vi "log analysis_gps.vi"() -> ()   [LabVIEW 2019] (continued)
,0*ce1f2ed1\n\t", "DUALANTENNAHEADINGA,USB3,0,53.0,FINESTEERING,2107,282441.200,02000000,d426,15824;SOL_COMPUTED,L1_FLOAT,-1.000000000,98.119506836,-70.068420410,0.0,360.000000000,180.000000000,\"631T\",15,6,6,6,04,00,20,02*34737370\n\t", "INSPVAXA,USB3,0,53.0,FINESTEERING,2107,282441.700,02000000,471d,15824;INS_ALIGNMENT_COMPLETE,INS_RTKFIXED,37.37044907161,126.72457798223,11.5726,22.3000,-0.1948,0.2179,0.0112,0.019648441,1.409240811,126.353403085,0.4397,0.2935,0.5431,0.1139,0.0925,0.0768,0.1391,0.1441,5.0591,0f000001,0*4c7348f3\n\t", "DUALANTENNAHEADINGA,USB3,0,53.0,FINESTEERING,2107,282442.200,02000000,d426,15824;SOL_COMPUTED,L1_FLOAT,-1.000000000,135.735549927,-62.905853271,0.0,360.000000000,180.000000000,\"631T\",15,6,6,6,04,00,20,02*7d1a323e\n\t", "DUALANTENNAHEADINGA,USB3,0,53.0,FINESTEERING,2107,282442.700,02000000,d426,15824;SOL_COMPUTED,L1_FLOAT,-1.000000000,139.850036621,-63.364013672,0.0,360.000000000,180.000000000,\"631T\",16,6,6,6,04,00,20,02*201824d6\n\t", "INSPVAXA,USB3,0,51.0,FINESTEERING,2107,282443.200,02000000,471d,15824;INS_ALIGNMENT_COMPLETE,INS_RTKFIXED,37.37044646413,126.72458151712,11.5864,22.3000,-0.1973,0.2015,0.0164,-0.221608077,1.394071169,127.627895652,0.4382,0.2942,0.5425,0.1139,0.0929,0.0768,0.1390,0.1440,5.0619,0f000001,0*d0821dfc\n\t", "DUALANTENNAHEADINGA,USB3,0,51.0,FINESTEERING,2107,282443.700,02000000,d426,15824;SOL_COMPUTED,NARROW_FLOAT,-1.000000000,112.599952698,-57.933044434,0.0,360.000000000,180.000000000,\"631T\",15,6,6,6,04,00,20,03*0a41350b\n\t", "DUALANTENNAHEADINGA,USB3,0,52.5,FINESTEERING,2107,282444.200,02000000,d426,15824;SOL_COMPUTED,L1_FLOAT,-1.000000000,94.401931763,-65.202850342,0.0,360.000000000,180.000000000,\"631T\",17,6,6,6,04,00,20,03*e210f1e8\n\t", "INSPVAXA,USB3,0,52.5,FINESTEERING,2107,282444.700,02000000,471d,15824;INS_ALIGNMENT_COMPLETE,INS_RTKFIXED,37.37044378367,126.72458489519,11.6040,22.3000,-0.1971,0.2104,0.0118,-0.197880099,2.000562987,128.752453378,0.4375,0.2942,0.5421,0.1140,0.0930,0.0767,0.1389,0.1439,5.0634,0f000001,0*c33b9934\n\t", "INSPVAXA,USB3,0,52.0,FINESTEERING,2107,282445.200,02000000,471d,15824;INS_ALIGNMENT_COMPLETE,INS_RTKFIXED,37.37044286692,126.72458603367,11.6088,22.3000,-0.1958,0.2105,0.0125,-0.182257004,1.882197193,129.119511082,0.4372,0.2942,0.5419,0.1140,0.0930,0.0767,0.1387,0.1438,5.0651,0f000001,0*e6286548\n\t", "INSPVAXA,USB3,0,52.0,FINESTEERING,2107,282445.700,02000000,471d,15824;INS_ALIGNMENT_COMPLETE,INS_RTKFIXED,37.37044196596,126.72458716165,11.6139,22.3000,-0.1860,0.1986,0.0135,-0.288793449,1.691261499,129.571848658,0.4372,0.2942,0.5419,0.1140,0.0930,0.0767,0.1387,0.1438,5.0651,0f000001,0*93ea3f3c\n\t", "INSPVAXA,USB3,0,49.5,FINESTEERING,2107,282446.200,02000000,471d,15824;INS_ALIGNMENT_COMPLETE,INS_RTKFIXED,37.37044104802,126.72458827290,11.6191,22.3000,-0.2036,0.2086,0.0326,-0.314944845,1.597002545,130.029060418,0.4370,0.2950,0.5417,0.1141,0.0931,0.0767,0.1386,0.1437,5.0666,0f000001,0*166a3618\n\t", "DUALANTENNAHEADINGA,USB3,0,49.5,FINESTEERING,2107,282446.700,02000000,d426,15824;SOL_COMPUTED,L1_FLOAT,-1.000000000,72.571334839,-68.740661621,0.0,360.000000000,180.000000000,\"631T\",16,6,6,6,04,00,20,02*f8abca53\n\t", "DUALANTENNAHEADINGA,USB3,0,51.0,FINESTEERING,2107,282447.200,02000000,d426,15824;SOL_COMPUTED,L1_FLOAT,-1.000000000,47.042289734,-21.824493408,0.0,80.520454407,171.226654053,\"631T\",17,6,6,6,04,00,20,02*c2df237f\n\t", "DUALANTENNAHEADINGA,USB3,0,51.0,FINESTEERING,2107,282447.700,02000000,d426,15824;SOL_COMPUTED,L1_FLOAT,-1.000000000,47.179916382,-22.115081787,0.0,81.568397522,172.185485840,\"631T\",16,6,6,6,04,00,20,02*ed165946\n\t", "DUALANTENNAHEADINGA,USB3,0,50.0,FINESTEERING,2107,282448.200,02000000,d426,15824;SOL_COMPUTED,L1_FLOAT,-1.000000000,62.731056213,-70.065948486,0.0,206.330291748,71.296012878,\"631T\",14,6,6,6,04,00,20,02*363416aa\n\t", "DUALANTENNAHEADINGA,USB3,0,50.0,FINESTEERING,2107,282448.700,02000000,d426,15824;SOL_COMPUTED,L1_FLOAT,-1.000000000,63.022411346,-70.363861084,0.0,209.852844238,71.028411865,\"631T\",14,6,6,6,04,00,20,02*916b79b1\n\t", "INSPVAXA,USB3,0,52.0,FINESTEERING,2107,282449.200,02000000,471d,15824;INS_ALIGNMENT_COMPLETE,INS_RTKFIXED,37.37043526808,126.72459474033,11.6436,22.3000,-0.2045,0.1792,0.0240,0.090566175,1.487884690,132.369305266,0.4363,0.2959,0.5410,0.1143,0.0932,0.0767,0.1382,0.1433,5.0710,0f000001,0*e0923cb2\n\t", "DUALANTENNAHEADINGA,USB3,0,52.0,FINESTEERING,2107,282449.700,02000000,d426,15824;SOL_COMPUTED,L1_FLOAT,-1.000000000,47.736373901,-41.870452881,0.0,87.065238953,101.863716125,\"631T\",13,6,6,6,04,00,20,02*14df9d16\n\t", "DUALANTENNAHEADINGA,USB3,0,53.5,FINESTEERING,2107,282450.200,02000000,d426,15824;SOL_COMPUTED,L1_FLOAT,-1.000000000,51.328735352,-27.176086426,0.0,71.032249451,148.623870850,\"631T\",13,6,6,6,04,00,20,02*70d3e876\n\t", "DUALANTENNAHEADINGA,USB3,0,53.5,FINESTEERING,2107,282450.700,02000000,d426,15824;SOL_COMPUTED,L1_FLOAT,-1.000000000,51.277191162,-27.081176758,0.0,70.920402527,148.848937988,\"631T\",13,6,6,6,04,00,20,02*7b58cb2d\n\t", "DUALANTENNAHEADINGA,USB3,0,52.5,FINESTEERING,2107,282451.200,02000000,d426,15824;SOL_COMPUTED,L1_FLOAT,-1.000000000,57.890838623,-57.911682129,0.0,124.624069214,87.193580627,\"631T\",15,6,6,6,04,00,20,02*079d44e7\n\t", "DUALANTENNAHEADINGA,USB3,0,52.5,FINESTEERING,2107,282451.700,02000000,d426,15824;SOL_COMPUTED,L1_FLOAT,-1.000000000,57.663475037,-57.904479980,0.0,124.210479736,87.412086487,\"631T\",14,6,6,6,04,00,20,03*cca5b843\n\t", "DUALANTENNAHEADINGA,USB3,0,52.0,FINESTEERING,2107,282452.200,02000000,d426,15824;SOL_COMPUTED,L1_FLOAT,-1.000000000,54.869430542,-44.105773926,0.0,97.000511169,118.565223694,\"631T\",14,6,6,6,04,00,20,02*875da1f2\n\t", "DUALANTENNAHEADINGA,USB3,0,52.0,FINESTEERING,2107,282452.700,02000000,d426,15824;SOL_COMPUTED,L1_FLOAT,-1.000000000,55.240604401,-44.770904541,0.0,98.983810425,117.544937134,\"631T\",14,6,6,6,04,00,20,02*e9f54d5e\n\t", "DUALANTENNAHEADINGA,USB3,0,50.5,FINESTEERING,2107,282453.200,02000000,d426,15824;SOL_COMPUTED,L1_FLOAT,-1.000000000,53.051345825,-30.869628906,0.0,85.964683533,159.088867188,\"631T\",12,6,6,6,04,00,20,02*9757b4ba\n\t", "DUALANTENNAHEADINGA,USB3,0,50.5,FINESTEERING,2107,282453.700,02000000,d426,15824;SOL_COMPUTED,L1_FLOAT,-1.000000000,53.156692505,-31.481872559,0.0,86.806381226,157.845855713,\"631T\",12,6,6,6,04,00,20,02*cbe10416\n\t", "DUALANTENNAHEADINGA,USB3,0,52.0,FINESTEERING,2107,282454.200,02000000,d426,15824;SOL_COMPUTED,L1_FLOAT,-1.000000000,52.780334473,-53.877258301,0.0,130.208221436,141.251815796,\"631T\",14,6,6,6,04,00,20,02*fcced73a\n\t", "DUALANTENNAHEADINGA,USB3,0,52.0,FINESTEERING,2107,282454.700,02000000,d426,15824;SOL_COMPUTED,L1_FLOAT,-1.000000000,52.636894226,-53.647705078,0.0,129.656005859,142.158767700,\"631T\",13,6,6,6,04,00,20,02*0d3c93fe\n\t", "DUALANTENNAHEADINGA,USB3,0,51.5,FINESTEERING,2107,282455.700,02000000,d426,15824;SOL_COMPUTED,L1_FLOAT,-1.000000000,51.760696411,-51.082702637,0.0,133.844039917,173.444122314,\"631T\",14,6,6,6,04,00,20,02*f8aac9e6\n\t", "DUALANTENNAHEADINGA,USB3,0,53.5,FINESTEERING,2107,282456.200,02000000,d426,15824;SOL_COMPUTED,L1_FLOAT,-1.000000000,51.028530121,-49.821136475,0.0,115.512840271,104.671615601,\"631T\",14,6,6,6,04,00,20,02*e59d7854\n\t", "DUALANTENNAHEADINGA,USB3,0,53.5,FINESTEERING,2107,282456.700,02000000,d426,15824;SOL_COMPUTED,L1_FLOAT,-1.000000000,51.237274170,-50.023620605,0.0,116.616584778,104.545890808,\"631T\",13,6,6,6,04,00,20,02*1b2f8a7d\n\t", "DUALANTENNAHEADINGA,USB3,0,53.0,FINESTEERING,2107,282457.200,02000000,d426,15824;SOL_COMPUTED,L1_FLOAT,-1.000000000,50.694931030,-44.774475098,0.0,121.998092651,121.907302856,\"631T\",13,6,6,6,04,00,20,02*d464c5aa\n\t", "DUALANTENNAHEADINGA,USB3,0,53.0,FINESTEERING,2107,282457.700,02000000,d426,15824;SOL_COMPUTED,L1_FLOAT,-1.000000000,50.592933655,-45.348266602,0.0,122.468826294,120.254112244,\"631T\",13,6,6,6,04,00,20,02*d8abe33e\n\t", "DUALANTENNAHEADINGA,USB3,0,53.0,FINESTEERING,2107,282458.200,02000000,d426,15824;SOL_COMPUTED,L1_FLOAT,-1.000000000,49.797100067,-45.644378662,0.0,104.331756592,110.018707275,\"631T\",15,6,6,6,04,00,20,02*7b675054\n\t", "DUALANTENNAHEADINGA,USB3,0,53.0,FINESTEERING,2107,282458.700,02000000,d426,15824;SOL_COMPUTED,L1_FLOAT,-1.000000000,50.209892273,-46.350616455,0.0,106.050132751,108.550285339,\"631T\",15,6,6,6,04,00,20,02*c27fecdc\n\t", "DUALANTENNAHEADINGA,USB3,0,49.5,FINESTEERING,2107,282459.200,02000000,d426,15824;SOL_COMPUTED,L1_FLOAT,-1.000000000,51.845520020,-58.692413330,0.0,123.868484497,115.955833435,\"631T\",15,5,5,5,04,00,20,03*67457323\n\t", "DUALANTENNAHEADINGA,USB3,0,49.5,FINESTEERING,2107,282459.700,02000000,d426,15824;SOL_COMPUTED,L1_FLOAT,-1.000000000,51.464805603,-60.732208252,0.0,125.312278748,109.238609314,\"631T\",15,5,5,5,04,00,20,02*8c6ba398\n\t", "DUALANTENNAHEADINGA,USB3,0,50.0,FINESTEERING,2107,282460.700,02000000,d426,15824;SOL_COMPUTED,L1_FLOAT,-1.000000000,54.102706909,-60.343048096,0.0,154.762100220,135.056198120,\"631T\",14,6,6,6,04,00,20,02*46d0133e\n\t", "DUALANTENNAHEADINGA,USB3,0,51.0,FINESTEERING,2107,282461.200,02000000,d426,15824;SOL_COMPUTED,L1_FLOAT,-1.000000000,54.517234802,-56.248260498,0.0,106.436035156,86.120704651,\"631T\",12,6,6,6,04,00,20,02*7e772430\n\t", "DUALANTENNAHEADINGA,USB3,0,53.0,FINESTEERING,2107,282462.200,02000000,d426,15824;SOL_COMPUTED,L1_FLOAT,-1.000000000,48.982975006,-50.048645020,0.0,87.434806824,84.797714233,\"631T\",12,6,6,6,04,00,20,02*0529a78d\n\t", "DUALANTENNAHEADINGA,USB3,0,53.0,FINESTEERING,2107,282462.700,02000000,d426,15824;SOL_COMPUTED,L1_FLOAT,-1.000000000,49.117179871,-50.247711182,0.0,88.570533752,85.136001587,\"631T\",13,6,6,6,04,00,20,03*84c2d42f\n\t", "DUALANTENNAHEADINGA,USB3,0,54.0,FINESTEERING,2107,282463.700,02000000,d426,15824;SOL_COMPUTED,L1_FLOAT,-1.000000000,51.500408173,-54.802459717,0.0,108.538322449,83.711227417,\"631T\",15,6,6,6,04,00,20,02*3dcbf296\n\t", "DUALANTENNAHEADINGA,USB3,0,51.5,FINESTEERING,2107,282465.200,02000000,d426,15824;SOL_COMPUTED,NARROW_FLOAT,-1.000000000,56.702713013,-55.800750732,0.0,137.773193359,136.991073608,\"631T\",13,6,6,6,04,00,20,03*fede75fb\n\t", "DUALANTENNAHEADINGA,USB3,0,49.5,FINESTEERING,2107,282466.200,02000000,d426,15824;SOL_COMPUTED,L1_FLOAT,-1.000000000,50.215934753,-52.944305420,0.0,107.166450500,95.447196960,\"631T\",15,6,6,6,04,00,20,02*0a3eeb82\n\t", "INSPVAXA,USB3,0,49.5,FINESTEERING,2107,282467.250,02000000,471d,15824;INS_ALIGNMENT_COMPLETE,INS_RTKFIXED,37.37040027529,126.72463299399,11.7361,22.3000,-0.1940,0.1986,-0.0035,0.679971609,0.798971146,127.016292493,0.4355,0.2951,0.5412,0.1133,0.0928,0.0767,0.1368,0.1419,5.0947,0f000001,0*9f6381ee\n\t", "DUALANTENNAHEADINGA,USB3,0,49.5,FINESTEERING,2107,282467.700,02000000,d426,15824;SOL_COMPUTED,L1_FLOAT,-1.000000000,52.617862701,-51.723999023,0.0,138.564620972,121.129493713,\"631T\",15,6,6,6,04,00,20,02*1b74d979\n\t", "DUALANTENNAHEADINGA,USB3,0,52.5,FINESTEERING,2107,282468.200,02000000,d426,15824;SOL_COMPUTED,L1_FLOAT,-1.000000000,53.229724884,-52.106597900,0.0,138.289840698,109.253112793,\"631T\",16,6,6,6,04,00,20,02*279e2280\n\t", "DUALANTENNAHEADINGA,USB3,0,51.5,FINESTEERING,2107,282469.200,02000000,d426,15824;SOL_COMPUTED,L1_FLOAT,-1.000000000,53.708850861,-50.439453125,0.0,142.785049438,121.784484863,\"631T\",13,6,6,6,04,00,20,02*6a3bd9b0\n\t", "DUALANTENNAHEADINGA,USB3,0,52.0,FINESTEERING,2107,282470.200,02000000,d426,15824;SOL_COMPUTED,L1_FLOAT,-1.000000000,64.190452576,-66.300750732,0.0,248.333297729,180.000000000,\"631T\",12,6,6,6,04,00,20,02*9fcca8a8\n\t", "INSPVAXA,USB3,0,52.0,FINESTEERING,2107,282470.750,02000000,471d,15824;INS_ALIGNMENT_COMPLETE,INS_RTKFIXED,37.37039399952,126.72464125042,11.7560,22.3000,-0.1944,0.2055,0.0095,0.556382070,0.833580794,124.571491117,0.4368,0.2954,0.5421,0.1138,0.0931,0.0768,0.1367,0.1417,5.0972,0f000001,0*6c9732d6\n\t", "DUALANTENNAHEADINGA,USB3,0,53.0,FINESTEERING,2107,282471.200,02000000,d426,15824;SOL_COMPUTED,NARROW_FLOAT,-1.000000000,77.375328064,-72.297668457,0.0,360.000000000,180.000000000,\"631T\",16,6,6,6,04,00,20,03*599578cb\n\t", "DUALANTENNAHEADINGA,USB3,0,46.5,FINESTEERING,2107,282472.200,02000000,d426,15824;SOL_COMPUTED,L1_FLOAT,-1.000000000,54.732860565,-45.831329346,0.0,98.283119202,178.546401978,\"631T\",13,7,7,7,04,00,20,02*8ccffb99\n\t", "DUALANTENNAHEADINGA,USB3,0,46.5,FINESTEERING,2107,282472.700,02000000,d426,15824;SOL_COMPUTED,L1_FLOAT,-1.000000000,54.959995270,-45.596282959,0.0,98.333869934,179.821563721,\"631T\",13,7,7,7,04,00,20,02*00d3f37b\n\t", "INSPVAXA,USB3,0,52.0,FINESTEERING,2107,282473.250,02000000,471d,15824;INS_ALIGNMENT_COMPLETE,INS_RTKFIXED,37.37038981275,126.72464739191,11.7746,22.3000,-0.1948,0.2277,0.0045,0.156747113,1.075368694,121.414050270,0.4373,0.2954,0.5425,0.1142,0.0935,0.0768,0.1366,0.1413,5.0978,0f000001,0*e88bca5a\n\t", "INSPVAXA,USB3,0,52.0,FINESTEERING,2107,282473.750,02000000,471d,15824;INS_ALIGNMENT_COMPLETE,INS_RTKFIXED,37.37038901794,126.72464863796,11.7783,22.3000,-0.1909,0.2328,0.0045,0.039175910,1.239409114,120.698239025,0.4373,0.2954,0.5425,0.1142,0.0935,0.0768,0.1366,0.1413,5.0978,0f000001,0*6f6aad10\n\t", "INSPVAXA,USB3,0,52.5,FINESTEERING,2107,282474.250,02000000,471d,15824;INS_ALIGNMENT_COMPLETE,INS_RTKFIXED,37.37038821663,126.72464993203,11.7822,22.3000,-0.1900,0.2213,-0.0032,0.050457416,1.361079347,119.957675424,0.4373,0.2953,0.5423,0.1143,0.0936,0.0767,0.1365,0.1412,5.0971,0f000001,0*04eefe7e\n\t", "DUALANTENNAHEADINGA,USB3,0,52.5,FINESTEERING,2107,282474.700,02000000,d426,15824;SOL_COMPUTED,NARROW_FLOAT,-1.000000000,53.444328308,-36.252197266,0.0,99.495506287,180.000000000,\"631T\",13,7,7,7,04,00,20,03*a63b34b7\n\t", "INSPVAXA,USB3,0,51.0,FINESTEERING,2107,282475.750,02000000,471d,15824;INS_ALIGNMENT_COMPLETE,INS_RTKFIXED,37.37038590363,126.72465390655,11.7950,22.3000,-0.1808,0.2394,-0.0047,0.109913426,1.377387594,117.860298903,0.4381,0.2954,0.5423,0.1145,0.0936,0.0767,0.1364,0.1410,5.0959,0f000001,0*7de89cb0\n\t", "DUALANTENNAHEADINGA,USB3,0,51.5,FINESTEERING,2107,282476.200,02000000,d426,15824;SOL_COMPUTED,L1_FLOAT,-1.000000000,55.533638000,-0.375610352,0.0,117.860015869,180.000000000,\"631T\",14,7,7,7,04,00,20,02*d327ff6e\n\t", "INSPVAXA,USB3,0,51.5,FINESTEERING,2107,282476.750,02000000,471d,15824;INS_ALIGNMENT_COMPLETE,INS_RTKFIXED,37.37038443010,126.72465662645,11.8037,22.3000,-0.1744,0.2321,0.0038,0.098053038,1.110033651,116.595542201,0.4382,0.2952,0.5423,0.1147,0.0936,0.0767,0.1363,0.1408,5.0950,0f000001,0*ea8caedb\n\t", "INSPVAXA,USB3,0,52.0,FINESTEERING,2107,282477.250,02000000,471d,15824;INS_ALIGNMENT_COMPLETE,INS_RTKFIXED,37.37038371373,126.72465798496,11.8086,22.3000,-0.1784,0.2376,0.0072,0.132722378,1.123390738,116.043560691,0.4382,0.2951,0.5421,0.1149,0.0937,0.0767,0.1362,0.1405,5.0949,0f000001,0*a21a9ce6\n\t", "DUALANTENNAHEADINGA,USB3,0,47.5,FINESTEERING,2107,282478.200,02000000,d426,15824;SOL_COMPUTED,NARROW_FLOAT,-1.000000000,53.676605225,18.221975327,0.0,112.330833435,180.000000000,\"631T\",17,7,7,7,04,00,20,03*123ff075\n\t", "INSPVAXA,USB3,0,47.5,FINESTEERING,2107,282478.750,02000000,471d,15824;INS_ALIGNMENT_COMPLETE,INS_RTKFIXED,37.37038162641,126.72466209113,11.8198,22.3000,-0.1768,0.2383,-0.0098,0.146556317,1.371576994,114.526516784,0.4387,0.2951,0.5427,0.1151,0.0939,0.0768,0.1361,0.1403,5.0955,0f000001,0*9c50f9d9\n\t", "DUALANTENNAHEADINGA,USB3,0,50.0,FINESTEERING,2107,282479.200,02000000,d426,15824;SOL_COMPUTED,NARROW_FLOAT,-1.000000000,51.679660797,16.235267639,0.0,131.237731934,180.000000000,\"631T\",15,7,7,7,04,00,20,03*76498f9b\n\t", "INSPVAXA,USB3,0,50.0,FINESTEERING,2107,282479.750,02000000,471d,15824;INS_ALIGNMENT_COMPLETE,INS_RTKFIXED,37.37038033615,126.72466486857,11.8253,22.3000,-0.1778,0.2630,-0.0031,-0.080326690,1.236523677,113.540262033,0.4414,0.2959,0.5454,0.1157,0.0941,0.0769,0.1359,0.1401,5.0966,0f000001,0*bc5588b9\n\t", "INSPVAXA,USB3,0,51.0,FINESTEERING,2107,282480.750,02000000,471d,15824;INS_ALIGNMENT_COMPLETE,INS_RTKFIXED,37.37037910395,126.72466763539,11.8294,22.3000,-0.1682,0.2496,-0.0083,-0.123932791,1.123250163,112.586404178,0.4418,0.2960,0.5463,0.1157,0.0942,0.0770,0.1357,0.1398,5.0977,0f000001,0*a24ca24f\n\t", "INSPVAXA,USB3,0,49.5,FINESTEERING,2107,282481.750,02000000,471d,15824;INS_ALIGNMENT_COMPLETE,INS_RTKFIXED,37.37037789694,126.72467048931,11.8351,22.3000,-0.1461,0.2327,0.0043,-0.310804253,1.123961293,111.895191809,0.4415,0.2959,0.5463,0.1157,0.0942,0.0769,0.1355,0.1395,5.0988,0f000001,0*973dff57\n\t", "INSPVAXA,USB3,0,50.5,FINESTEERING,2107,282482.250,02000000,471d,15824;INS_ALIGNMENT_COMPLETE,INS_RTKFIXED,37.37037731116,126.72467190347,11.8384,22.3000,-0.1477,0.2523,-0.0105,-0.265666832,1.108878256,111.633485530,0.4404,0.2956,0.5456,0.1156,0.0941,0.0769,0.1353,0.1392,5.0999,0f000001,0*cd6558ee\n\t", "INSPVAXA,USB3,0,50.5,FINESTEERING,2107,282482.750,02000000,471d,15824;INS_ALIGNMENT_COMPLETE,INS_RTKFIXED,37.37037674280,126.72467330399,11.8420,22.3000,-0.1430,0.2494,-0.0020,-0.174444219,1.137466494,111.346444953,0.4404,0.2956,0.5456,0.1156,0.0941,0.0769,0.1353,0.1392,5.0999,0f000001,0*2a49352f\n\t", "INSPVAXA,USB3,0,50.0,FINESTEERING,2107,282483.250,02000000,471d,15824;INS_ALIGNMENT_COMPLETE,INS_RTKFIXED,37.37037616883,126.72467474324,11.8449,22.3000,-0.1483,0.2627,-0.0049,-0.159355428,1.028327028,111.093660255,0.4396,0.2956,0.5446,0.1155,0.0941,0.0768,0.1351,0.1389,5.1012,0f000001,0*e9226b16\n\t", "INSPVAXA,USB3,0,50.0,FINESTEERING,2107,282483.750,02000000,471d,15824;INS_ALIGNMENT_COMPLETE,INS_RTKFIXED,37.37037559924,126.72467616191,11.8460,22.3000,-0.1456,0.2485,-0.0071,-0.147252002,0.996738159,110.847183596,0.4396,0.2956,0.5446,0.1155,0.0941,0.0768,0.1351,0.1389,5.1012,0f000001,0*6063b49d\n\t", "INSPVAXA,USB3,0,51.5,FINESTEERING,2107,282484.750,02000000,471d,15824;INS_ALIGNMENT_COMPLETE,INS_RTKFIXED,37.37037448665,126.72467902626,11.8522,22.3000,-0.1407,0.2484,-0.0090,-0.064873099,1.145438573,110.168729835,0.4390,0.2955,0.5438,0.1153,0.0940,0.0767,0.1348,0.1386,5.1026,0f000001,0*a0636209\n\t", "INSPVAXA,USB3,0,51.0,FINESTEERING,2107,282485.250,02008000,471d,15824;INS_ALIGNMENT_COMPLETE,INS_RTKFIXED,37.37037393424,126.72468050363,11.8549,22.3000,-0.1324,0.2566,-0.0083,0.002695886,0.976355436,109.894464634,0.4390,0.2956,0.5434,0.1153,0.0939,0.0767,0.1346,0.1383,5.1041,0f000001,0*d70e669a\n\t", "INSPVAXA,USB3,0,51.0,FINESTEERING,2107,282485.750,02008000,471d,15824;INS_ALIGNMENT_COMPLETE,INS_RTKFIXED,37.37037339561,126.72468193841,11.8561,22.3000,-0.1291,0.2465,-0.0040,0.117309078,0.863917654,109.567582429,0.4390,0.2956,0.5434,0.1153,0.0939,0.0767,0.1346,0.1383,5.1041,0f000001,0*167aa476\n\t", "DUALANTENNAHEADINGA,USB3,0,52.0,FINESTEERING,2107,282486.200,02008000,d426,15824;SOL_COMPUTED,L1_FLOAT,-1.000000000,124.986564636,-52.100769043,0.0,360.000000000,180.000000000,\"631T\",12,6,6,6,04,00,20,02*25d98b4c\n\t", "INSPVAXA,USB3,0,52.0,FINESTEERING,2107,282486.750,02008000,471d,15824;INS_ALIGNMENT_COMPLETE,INS_RTKFIXED,37.37037231578,126.72468487356,11.8580,22.3000,-0.1363,0.2539,-0.0079,0.065083536,0.658526684,108.961373177,0.4389,0.2956,0.5429,0.1152,0.0940,0.0767,0.1344,0.1380,5.1058,0f000001,0*795b201f\n\t", "INSPVAXA,USB3,0,53.0,FINESTEERING,2107,282487.750,02008000,471d,15824;INS_ALIGNMENT_COMPLETE,INS_RTKFIXED,37.37037124612,126.72468781330,11.8615,22.3000,-0.1351,0.2529,-0.0014,0.028036761,0.509941288,108.259170524,0.4390,0.2956,0.5427,0.1151,0.0939,0.0767,0.1342,0.1378,5.1072,0f000001,0*7116cc62\n\t", "INSPVAXA,USB3,0,50.5,FINESTEERING,2107,282488.750,02008000,471d,15824;INS_ALIGNMENT_COMPLETE,INS_RTKFIXED,37.37037023523,126.72469074006,11.8656,22.3000,-0.1204,0.2670,0.0002,0.044873893,0.831014389,107.580535120,0.4389,0.2956,0.5425,0.1150,0.0937,0.0767,0.1339,0.1375,5.1082,0f000001,0*4cab4b69\n\t", "INSPVAXA,USB3,0,51.0,FINESTEERING,2107,282489.250,02000000,471d,15824;INS_ALIGNMENT_COMPLETE,INS_RTKFIXED,37.37036974630,126.72469219938,11.8668,22.3000,-0.1082,0.2562,0.0055,0.037042210,0.796968035,107.199262674,0.4392,0.2956,0.5428,0.1149,0.0936,0.0767,0.1337,0.1373,5.1092,0f000001,0*9fc09916\n\t", "INSPVAXA,USB3,0,52.0,FINESTEERING,2107,282490.250,02000000,471d,15824;INS_ALIGNMENT_COMPLETE,INS_RTKFIXED,37.37036877450,126.72469515177,11.8697,22.3000,-0.1086,0.2580,0.0081,-0.074758775,1.106093430,106.454761549,0.4393,0.2955,0.5430,0.1148,0.0934,0.0768,0.1335,0.1371,5.1102,0f000001,0*37127645\n\t", "INSPVAXA,USB3,0,52.0,FINESTEERING,2107,282490.750,02000000,471d,15824;INS_ALIGNMENT_COMPLETE,INS_RTKFIXED,37.37036829389,126.72469663971,11.8737,22.3000,-0.1049,0.2625,0.0062,-0.116881471,1.024892331,106.058307514,0.4393,0.2955,0.5430,0.1148,0.0934,0.0768,0.1335,0.1371,5.1102,0f000001,0*7841381f\n\t", "INSPVAXA,USB3,0,51.5,FINESTEERING,2107,282491.250,02000000,471d,15824;INS_ALIGNMENT_COMPLETE,INS_RTKFIXED,37.37036783071,126.72469814477,11.8773,22.3000,-0.1005,0.2703,0.0019,-0.302758145,0.967035823,105.571562776,0.4390,0.2953,0.5427,0.1146,0.0933,0.0767,0.1334,0.1370,5.1117,0f000001,0*df8a40e1\n\t", "INSPVAXA,USB3,0,53.0,FINESTEERING,2107,282492.250,02000000,471d,15824;INS_ALIGNMENT_COMPLETE,INS_RTKFIXED,37.37036690492,126.72470114805,11.8868,22.3000,-0.1128,0.2686,-0.0005,-0.341749532,1.011987346,104.657671438,0.4386,0.2951,0.5424,0.1145,0.0933,0.0767,0.1332,0.1368,5.1133,0f000001,0*36e30592\n\t", "INSPVAXA,USB3,0,53.0,FINESTEERING,2107,282492.750,02000000,471d,15824;INS_ALIGNMENT_COMPLETE,INS_RTKFIXED,37.37036645131,126.72470265161,11.8901,22.3000,-0.1035,0.2695,-0.0047,-0.206753293,0.813426880,104.258109250,0.4386,0.2951,0.5424,0.1145,0.0933,0.0767,0.1332,0.1368,5.1133,0f000001,0*577226f1\n\t", "INSPVAXA,USB3,0,50.0,FINESTEERING,2107,282493.250,02000000,471d,15824;INS_ALIGNMENT_COMPLETE,INS_RTKFIXED,37.37036601456,126.72470416352,11.8919,22.3000,-0.1012,0.2672,-0.0093,-0.224228213,0.685864648,103.742995644,0.4383,0.2950,0.5422,0.1144,0.0932,0.0767,0.1331,0.1366,5.1149,0f000001,0*31397ff1\n\t", "INSPVAXA,USB3,0,50.0,FINESTEERING,2107,282493.750,02000000,471d,15824;INS_ALIGNMENT_COMPLETE,INS_RTKFIXED,37.37036559899,126.72470566002,11.8945,22.3000,-0.1067,0.2704,-0.0029,-0.332770610,0.803747172,103.266979310,0.4383,0.2950,0.5422,0.1144,0.0932,0.0767,0.1331,0.1366,5.1149,0f000001,0*9ccbb3e3\n\t", "INSPVAXA,USB3,0,54.0,FINESTEERING,2107,282494.250,02000000,471d,15824;INS_ALIGNMENT_COMPLETE,INS_RTKFIXED,37.37036518833,126.72470716061,11.8982,22.3000,-0.0992,0.2825,-0.0009,-0.390155029,0.844314939,102.750620694,0.4383,0.2950,0.5423,0.1144,0.0933,0.0767,0.1329,0.1365,5.1164,0f000001,0*37164162\n\t", "INSPVAXA,USB3,0,54.0,FINESTEERING,2107,282494.750,02000000,471d,15824;INS_ALIGNMENT_COMPLETE,INS_RTKFIXED,37.37036477713,126.72470868073,11.9009,22.3000,-0.0879,0.2706,0.0036,-0.341565952,0.784824904,102.134248180,0.4383,0.2950,0.5423,0.1144,0.0933,0.0767,0.1329,0.1365,5.1164,0f000001,0*6a9baff3\n\t", "INSPVAXA,USB3,0,52.0,FINESTEERING,2107,282495.750,02000000,471d,15824;INS_ALIGNMENT_COMPLETE,INS_RTKFIXED,37.37036401120,126.72471176105,11.9046,22.3000,-0.0834,0.2786,-0.0076,-0.308157155,0.761064852,100.941117040,0.4380,0.2949,0.5422,0.1143,0.0933,0.0767,0.1328,0.1363,5.1178,0f000001,0*054ad5c7\n\t", "INSPVAXA,USB3,0,50.5,FINESTEERING,2107,282496.250,02000000,471d,15824;INS_ALIGNMENT_COMPLETE,INS_RTKFIXED,37.37036364901,126.72471328274,11.9089,22.3000,-0.0739,0.2539,-0.0014,-0.343894984,0.754370105,100.232900120,0.4379,0.2949,0.5421,0.1143,0.0933,0.0767,0.1327,0.1362,5.1190,0f000001,0*8784bafb\n\t", "INSPVAXA,USB3,0,50.5,FINESTEERING,2107,282496.750,02000000,471d,15824;INS_ALIGNMENT_COMPLETE,INS_RTKFIXED,37.37036328787,126.72471481476,11.9136,22.3000,-0.0700,0.2693,-0.0009,-0.270371003,0.729660939,99.468887752,0.4379,0.2949,0.5421,0.1143,0.0933,0.0767,0.1327,0.1362,5.1190,0f000001,0*224a36a2\n\t", "INSPVAXA,USB3,0,52.0,FINESTEERING,2107,282497.250,02000000,471d,15824;INS_ALIGNMENT_COMPLETE,INS_RTKFIXED,37.37036295953,126.72471635660,11.9170,22.3000,-0.0692,0.2638,0.0039,-0.487791758,0.697577068,98.688104249,0.4380,0.2950,0.5422,0.1144,0.0934,0.0767,0.1326,0.1361,5.1201,0f000001,0*5983bd1e\n\t", "INSPVAXA,USB3,0,52.0,FINESTEERING,2107,282497.750,02000000,471d,15824;INS_ALIGNMENT_COMPLETE,INS_RTKFIXED,37.37036264142,126.72471787968,11.9197,22.3000,-0.0695,0.2760,-0.0054,-0.578412192,0.764831938,97.837503717,0.4380,0.2950,0.5422,0.1144,0.0934,0.0767,0.1326,0.1361,5.1201,0f000001,0*bf0827fb\n\t", "INSPVAXA,USB3,0,50.5,FINESTEERING,2107,282498.250,02000000,471d,15824;INS_ALIGNMENT_COMPLETE,INS_RTKFIXED,37.37036233909,126.72471942444,11.9220,22.3000,-0.0554,0.2842,0.0042,-0.538460345,0.850776558,96.860804388,0.4376,0.2949,0.5421,0.1145,0.0934,0.0767,0.1325,0.1359,5.1211,0f000001,0*e69b7700\n\t", "INSPVAXA,USB3,0,50.5,FINESTEERING,2107,282498.750,02000000,471d,15824;INS_ALIGNMENT_COMPLETE,INS_RTKFIXED,37.37036207253,126.72472096393,11.9246,22.3000,-0.0513,0.2714,0.0039,-0.548055416,0.760878793,95.595246784,0.4376,0.2949,0.5421,0.1145,0.0934,0.0767,0.1325,0.1359,5.1211,0f000001,0*75d334ae\n\t", "INSPVAXA,USB3,0,51.0,FINESTEERING,2107,282499.250,02000000,471d,15824;INS_ALIGNMENT_COMPLETE,INS_RTKFIXED,37.37036182665,126.72472251722,11.9274,22.3000,-0.0518,0.2707,0.0042,-0.612176508,0.765223252,94.525809257,0.4377,0.2950,0.5421,0.1146,0.0936,0.0767,0.1324,0.1357,5.1220,0f000001,0*ec8d0c0f\n\t", "INSPVAXA,USB3,0,51.0,FINESTEERING,2107,282499.750,02000000,471d,15824;INS_ALIGNMENT_COMPLETE,INS_RTKFIXED,37.37036160600,126.72472408768,11.9291,22.3000,-0.0494,0.2821,-0.0083,-0.781502529,0.706412197,93.339152024,0.4377,0.2950,0.5421,0.1146,0.0936,0.0767,0.1324,0.1357,5.1220,0f000001,0*d9b69855\n\t", "INSPVAXA,USB3,0,53.0,FINESTEERING,2107,282500.250,02000000,471d,15824;INS_ALIGNMENT_COMPLETE,INS_RTKFIXED,37.37036138755,126.72472565119,11.9317,22.3000,-0.0342,0.2702,0.0095,-0.593682831,0.623847561,91.416153722,0.4373,0.2951,0.5419,0.1148,0.0938,0.0767,0.1322,0.1355,5.1229,0f000001,0*07814bab\n\t", "INSPVAXA,USB3,0,53.0,FINESTEERING,2107,282500.750,02000000,471d,15824;INS_ALIGNMENT_COMPLETE,INS_RTKFIXED,37.37036130198,126.72472720567,11.9351,22.3000,0.0292,0.2886,0.0019,-0.781993907,0.527535072,86.351201750,0.4373,0.2951,0.5419,0.1148,0.0938,0.0767,0.1322,0.1355,5.1229,0f000001,0*6a6ac25a\n\t", "INSPVAXA,USB3,0,50.5,FINESTEERING,2107,282501.250,02000000,471d,15824;INS_ALIGNMENT_COMPLETE,INS_RTKFIXED,37.37036131745,126.72472879768,11.9390,22.3000,0.0369,0.2857,-0.0120,-0.997390809,0.433664742,81.039166738,0.4370,0.2954,0.5418,0.1155,0.0947,0.0767,0.1321,0.1353,5.1226,0f000001,0*2c9768ec\n\t", "INSPVAXA,USB3,0,50.5,FINESTEERING,2107,282501.750,02000000,471d,15824;INS_ALIGNMENT_COMPLETE,INS_RTKFIXED,37.37036141879,126.72473040754,11.9428,22.3000,0.0024,0.2788,-0.0052,-1.183204075,0.224327122,76.081887809,0.4370,0.2954,0.5418,0.1155,0.0947,0.0767,0.1321,0.1353,5.1226,0f000001,0*e82bc0a6\n\t", "INSPVAXA,USB3,0,52.5,FINESTEERING,2107,282502.250,02000000,471d,15824;INS_ALIGNMENT_COMPLETE,INS_RTKFIXED,37.37036164481,126.72473194519,11.9462,22.3000,0.0415,0.2803,0.0079,-1.160166771,-0.046948160,70.699699998,0.4369,0.2959,0.5417,0.1169,0.0967,0.0767,0.1320,0.1349,5.1194,0f000001,0*06dae310\n\t", "INSPVAXA,USB3,0,52.5,FINESTEERING,2107,282502.750,02000000,471d,15824;INS_ALIGNMENT_COMPLETE,INS_RTKFIXED,37.37036200144,126.72473343849,11.9497,22.3000,0.0229,0.2449,0.0184,-1.242261291,-0.215624383,65.570089717,0.4369,0.2959,0.5417,0.1169,0.0967,0.0767,0.1320,0.1349,5.1194,0f000001,0*37a9ba1d\n\t", "INSPVAXA,USB3,0,50.0,FINESTEERING,2107,282503.250,02000000,471d,15824;INS_ALIGNMENT_COMPLETE,INS_RTKFIXED,37.37036244144,126.72473485715,11.9546,22.3000,0.1159,0.2427,0.0087,-1.370274877,-0.522424319,60.146587364,0.4368,0.2966,0.5416,0.1192,0.0988,0.0767,0.1318,0.1345,5.1111,0f000001,0*9f9b3eba\n\t", "INSPVAXA,USB3,0,50.0,FINESTEERING,2107,282503.750,02000000,471d,15824;INS_ALIGNMENT_COMPLETE,INS_RTKFIXED,37.37036302784,126.72473625079,11.9579,22.3000,0.1573,0.2456,0.0068,-1.326431987,-0.638529875,54.895159113,0.4368,0.2966,0.5416,0.1192,0.0988,0.0767,0.1318,0.1345,5.1111,0f000001,0*c3a1e695\n\t", "INSPVAXA,USB3,0,51.0,FINESTEERING,2107,282504.250,02000000,471d,15824;INS_ALIGNMENT_COMPLETE,INS_RTKFIXED,37.37036369327,126.72473758611,11.9611,22.3000,0.1628,0.2237,0.0021,-1.236535008,-0.784458797,49.797084734,0.4377,0.2981,0.5419,0.1224,0.1023,0.0767,0.1314,0.1337,5.1002,0f000001,0*ce2dc0c6\n\t", "INSPVAXA,USB3,0,51.0,FINESTEERING,2107,282504.750,02000000,471d,15824;INS_ALIGNMENT_COMPLETE,INS_RTKFIXED,37.37036443928,126.72473881419,11.9655,22.3000,0.1771,0.2224,-0.0093,-1.091153284,-0.604631231,44.754867869,0.4377,0.2981,0.5419,0.1224,0.1023,0.0767,0.1314,0.1337,5.1002,0f000001,0*68fd2785\n\t", "INSPVAXA,USB3,0,51.0,FINESTEERING,2107,282505.250,02000000,471d,15824;INS_ALIGNMENT_COMPLETE,INS_RTKFIXED,37.37036527959,126.72473995022,11.9707,22.3000,0.1963,0.1952,-0.0121,-1.138350697,-0.474117376,39.571733238,0.4394,0.3003,0.5422,0.1267,0.1058,0.0767,0.1307,0.1325,5.0879,0f000001,0*6827ef91\n\t", "INSPVAXA,USB3,0,51.0,FINESTEERING,2107,282505.750,02000000,471d,15824;INS_ALIGNMENT_COMPLETE,INS_RTKFIXED,37.37036623616,126.72474098646,11.9763,22.3000,0.2120,0.1861,0.0048,-1.165263195,-0.362025094,34.418588384,0.4394,0.3003,0.5422,0.1267,0.1058,0.0767,0.1307,0.1325,5.0879,0f000001,0*40d9afbc\n\t", "INSPVAXA,USB3,0,51.5,FINESTEERING,2107,282506.250,02000000,471d,15824;INS_ALIGNMENT_COMPLETE,INS_RTKFIXED,37.37036720685,126.72474192456,11.9800,22.3000,0.2212,0.1614,0.0108,-1.132985321,-0.180413000,28.958926810,0.4417,0.3033,0.5424,0.1317,0.1100,0.0768,0.1296,0.1309,5.0779,0f000001,0*2e0d677d\n\t", "INSPVAXA,USB3,0,51.5,FINESTEERING,2107,282506.750,02000000,471d,15824;INS_ALIGNMENT_COMPLETE,INS_RTKFIXED,37.37036827241,126.72474279747,11.9819,22.3000,0.2642,0.1305,0.0010,-1.072910910,-0.236865707,23.702771649,0.4417,0.3033,0.5424,0.1317,0.1100,0.0768,0.1296,0.1309,5.0779,0f000001,0*c0c775a0\n\t", "INSPVAXA,USB3,0,51.0,FINESTEERING,2107,282507.250,02000000,471d,15824;INS_ALIGNMENT_COMPLETE,INS_RTKFIXED,37.37036943623,126.72474351475,11.9844,22.3000,0.2890,0.1143,0.0134,-1.116078326,-0.545577808,18.460028821,0.4448,0.3070,0.5424,0.1371,0.1144,0.0767,0.1279,0.1286,5.0714,0f000001,0*f2488cfe\n\t", "INSPVAXA,USB3,0,49.5,FINESTEERING,2107,282508.250,02000000,471d,15824;INS_ALIGNMENT_COMPLETE,INS_RTKFIXED,37.37036997810,126.72474418441,11.9888,22.3000,-0.0010,0.0343,0.0051,-0.948239100,-0.592787875,16.930139244,0.4486,0.3110,0.5423,0.1420,0.1207,0.0767,0.1255,0.1258,5.0683,0f000001,0*51dd059e\n\tsystem status\texception 2 28.000000 0 160\trobot status\t346.259842\t26.604893\t11.988800\t-0.948239\t-0.592788\t73.069861\t0.103000\t0.156000\n\t\n15:28:10.7\tlog_raw\tgps_raw\t#INSPVAXA,USB3,0,49.5,FINESTEERING,2107,282508.750,02000000,471d,15824;INS_ALIGNMENT_COMPLETE,INS_RTKFIXED,37.37036994386,126.72474436952,11.9909,22.3000,0.0056,0.0342,0.0053,-0.946500303,-0.592283051,16.912290627,0.4486,0.3110,0.5423,0.1420,0.1207,0.0767,0.1255,0.1258,5.0683,0f000001,0*09452605\n\tsystem status\texception 2 28.000000 0 160\trobot status\t346.276239\t26.601092\t11.990900\t-0.946500\t-0.592283\t73.087709\t0.103000\t0.156000\n\t\n15:28:11.2\tlog_raw\tgps_raw\t#INSPVAXA,USB3,0,51.0,FINESTEERING,2107,282509.250,02000000,471d,15824;INS_ALIGNMENT_COMPLETE,INS_RTKFIXED,37.37036993090,126.72474452786,11.9926,22.3000,0.0102,0.0361,0.0058,-0.944896447,-0.590729782,16.915447262,0.4529,0.3176,0.5421,0.1446,0.1223,0.0767,0.1224,0.1224,5.0667,0f000001,0*6e2fa647\n\tsystem status\texception 2 28.000000 0 160\trobot status\t346.290265\t26.599653\t11.992600\t-0.944896\t-0.590730\t73.084553\t0.103000\t0.156000\n\t\n15:28:11.7\tlog_raw\tgps_raw\t\tsystem status\texception 2 28.000000 0 160\trobot status\t346.301631\t26.601055\t11.993800\t-0.944236\t-0.592815\t73.083852\t0.103000\t0.156000\n\t\n15:28:12.2\tlog_raw\tgps_raw\t#INSPVAXA,USB3,0,53.0,FINESTEERING,2107,282510.250,02000000,471d,15824;INS_ALIGNMENT_COMPLETE,INS_RTKFIXED,37.37036996579,126.72474474686,11.9940,22.3000,0.0173,0.0357,0.0059,-0.945727300,-0.590701581,16.921367979,0.4568,0.3226,0.5419,0.1454,0.1213,0.0767,0.1190,0.1189,5.0583,0f000001,0*ffef94ef\n\tsystem status\texception 2 28.000000 0 160\trobot status\t346.309663\t26.603525\t11.994000\t-0.945727\t-0.590702\t73.078632\t0.103000\t0.156000\n\t\n15:28:12.7\tlog_raw\tgps_raw\t\tsystem status\texception 2 28.000000 0 160\trobot status\t346.313655\t26.606935\t11.993200\t-0.945766\t-0.586317\t73.066857\t0.103000\t0.156000\n\t\n15:28:13.2\tlog_raw\tgps_raw\t#INSPVAXA,USB3,0,52.5,FINESTEERING,2107,282511.250,02000000,471d,15824;INS_ALIGNMENT_COMPLETE,INS_RTKFIXED,37.37037004020,126.72474481545,11.9932,22.3000,0.0243,0.0321,0.0064,-0.946167296,-0.585921759,16.948767668,0.4597,0.3251,0.5417,0.1447,0.1186,0.0767,0.1156,0.1154,5.0445,0f000001,0*7b6abdb9\n\tsystem status\texception 2 28.000000 0 160\trobot status\t346.315739\t26.611783\t11.993200\t-0.946167\t-0.585922\t73.051232\t0.103000\t0.156000\n\t\n15:28:13.7\tlog_raw\tgps_raw\t#INSPVAXA,USB3,0,52.5,FINESTEERING,2107,282511.750,02000000,471d,15824;INS_ALIGNMENT_COMPLETE,INS_RTKFIXED,37.37037009329,126.72474481876,11.9942,22.3000,0.0266,0.0296,0.0059,-0.946113144,-0.582976087,16.966624089,0.4597,0.3251,0.5417,0.1447,0.1186,0.0767,0.1156,0.1154,5.0445,0f000001,0*617dc724\n\tsystem status\texception 2 28.000000 0 160\trobot status\t346.316032\t26.617675\t11.994200\t-0.946113\t-0.582976\t73.033376\t0.103000\t0.156000\n\t\n15:28:14.2\tlog_raw\tgps_raw\t#INSPVAXA,USB3,0,52.5,FINESTEERING,2107,282512.250,02000000,471d,15824;INS_ALIGNMENT_COMPLETE,INS_RTKFIXED,37.37037014737,126.72474480897,11.9952,22.3000,0.0300,0.0277,0.0058,-0.945767980,-0.581738683,16.984774160,0.4614,0.3254,0.5416,0.1426,0.1149,0.0767,0.1126,0.1124,5.0293,0f000001,0*18dcd093\n\tsystem status\texception 2 28.000000 0 160\trobot status\t346.315165\t26.623677\t11.995200\t-0.945768\t-0.581739\t73.015226\t0.103000\t0.156000\n\t\n15:28:14.7\tlog_raw\tgps_raw\t\tsystem status\texception 2 28.000000 0 160\trobot status\t346.313390\t26.629735\t11.996300\t-0.945482\t-0.578421\t72.995394\t0.103000\t0.156000\n\t\n15:28:15.2\tlog_raw\tgps_raw\t\tsystem status\texception 2 28.000000 0 160\trobot status\t346.310905\t26.635102\t11.997100\t-0.945925\t-0.578644\t72.975991\t0.103000\t0.156000\n\t\n15:28:15.7\tlog_raw\tgps_raw\t\tsystem status\texception 2 28.000000 0 160\trobot status\t346.307772\t26.639995\t11.997900\t-0.946669\t-0.578776\t72.958003\t0.103000\t0.156000\n\t\n15:28:16.2\tlog_raw\tgps_raw\t\tsystem status\texception 2 28.000000 0 160\trobot status\t346.304326\t26.644527\t11.998300\t-0.945581\t-0.576866\t72.939859\t0.103000\t0.156000\n\t\n15:28:16.7\tlog_raw\tgps_raw\t#INSPVAXA,USB3,0,50.5,FINESTEERING,2107,282514.750,02000000,471d,15824;INS_ALIGNMENT_COMPLETE,INS_RTKFIXED,37.37037037038,126.72474464474,11.9984,22.3000,0.0379,0.0170,0.0059,-0.942581332,-0.576970868,17.074319764,0.4609,0.3217,0.5415,0.1361,0.1072,0.0767,0.1082,0.1079,5.0056,0f000001,0*ba3ae658\n\t", "INSPVAXA,USB3,0,50.0,FINESTEERING,2107,282532.800,02000000,471d,15824;INS_ALIGNMENT_COMPLETE,INS_RTKFIXED,37.37036990032,126.72474422565,11.9691,22.3000,0.0075,0.0051,0.0018,-0.932116001,-0.549055451,17.452522918,0.2503,0.2036,0.3279,0.0447,0.0435,0.0399,0.0917,0.0916,4.9913,0f000005,0*47d3a519\n\tsystem status\texception 0 28.000000 0 60\trobot status\t346.263495\t26.596260\t11.969100\t-0.932116\t-0.549055\t72.547477\t0.097000\t0.019000\n\t\n15:28:35.3\tlog_raw\tgps_raw\t\tsystem status\texception 0 28.000000 0 60\trobot status\t346.259446\t26.587060\t11.968800\t-0.932260\t-0.546298\t72.538547\t0.097000\t0.019000\n\t\n15:28:35.8\tlog_raw\tgps_raw\t\tsystem status\texception 0 28.000000 0 60\trobot status\t346.258585\t26.585056\t11.968900\t-0.932112\t-0.548446\t72.536891\t0.097000\t0.019000\n\t\n15:28:36.3\tlog_raw\tgps_raw\t\tsystem status\texception 0 28.000000 0 60\trobot status\t346.258032\t26.583583\t11.969100\t-0.930409\t-0.549639\t72.534290\t0.097000\t0.019000\n\t\n15:28:36.8\tlog_raw\tgps_raw\t\t", "INSPVAXA,USB3,0,51.5,FINESTEERING,2107,282535.800,02000000,471d,15824;INS_ALIGNMENT_COMPLETE,INS_RTKFIXED,37.37036976834,126.72474416785,11.9702,22.3000,0.0056,0.0032,0.0025,-0.929895775,-0.548968401,17.475093869,0.2332,0.1853,0.3065,0.0346,0.0344,0.0316,0.0907,0.0908,4.9937,0f000005,0*4023dcd5\n\t", "INSPVAXA,USB3,0,50.0,FINESTEERING,2107,282539.300,02000000,471d,15824;INS_ALIGNMENT_COMPLETE,INS_RTKFIXED,37.37036978494,126.72474420325,11.9738,22.3000,0.0064,0.0050,0.0000,-0.929010849,-0.553956795,17.498282096,0.2195,0.1742,0.2911,0.0344,0.0343,0.0312,0.0907,0.0907,4.9970,0f000005,0*d5ca5fec\n\t", "INSPVAXA,USB3,0,50.0,FINESTEERING,2107,282539.800,02000000,471d,15824;INS_ALIGNMENT_COMPLETE,INS_RTKFIXED,37.37036978547,126.72474420294,11.9740,22.3000,0.0057,0.0046,-0.0006,-0.928135353,-0.553814797,17.500957060,0.2195,0.1742,0.2911,0.0344,0.0343,0.0312,0.0907,0.0907,4.9970,0f000005,0*764a2b63\n\t", "INSPVAXA,USB3,0,51.5,FINESTEERING,2107,282540.800,02000000,471d,15824;INS_ALIGNMENT_COMPLETE,INS_RTKFIXED,37.37036978786,126.72474420160,11.9749,22.3000,0.0059,0.0033,-0.0010,-0.930808234,-0.552950862,17.507619402,0.2170,0.1726,0.2881,0.0344,0.0343,0.0312,0.0907,0.0907,4.9979,0f000005,0*a62a7559\n\t", "INSPVAXA,USB3,0,52.0,FINESTEERING,2107,282541.300,02000000,471d,15824;INS_ALIGNMENT_COMPLETE,INS_RTKFIXED,37.37036978965,126.72474419874,11.9755,22.3000,0.0062,0.0033,-0.0009,-0.929974258,-0.549981203,17.509762902,0.2148,0.1713,0.2853,0.0344,0.0343,0.0312,0.0907,0.0906,4.9990,0f000005,0*bfdf10fc\n\t", "INSPVAXA,USB3,0,51.0,FINESTEERING,2107,282542.300,02000000,471d,15824;INS_ALIGNMENT_COMPLETE,INS_RTKFIXED,37.37036979234,126.72474420075,11.9765,22.3000,0.0055,0.0042,-0.0011,-0.931303287,-0.550383804,17.513004311,0.2130,0.1703,0.2828,0.0344,0.0343,0.0312,0.0907,0.0906,5.0000,0f000005,0*b690bd46\n\t", "INSPVAXA,USB3,0,47.5,FINESTEERING,2107,282543.300,02000000,471d,15824;INS_ALIGNMENT_COMPLETE,INS_RTKFIXED,37.37036978809,126.72474420745,11.9781,22.3000,0.0036,0.0055,-0.0013,-0.931308273,-0.552026668,17.515229582,0.2114,0.1694,0.2805,0.0344,0.0343,0.0312,0.0907,0.0906,5.0009,0f000005,0*ba0ef0aa\n\t", "INSPVAXA,USB3,0,47.5,FINESTEERING,2107,282543.800,02000000,471d,15824;INS_ALIGNMENT_COMPLETE,INS_RTKFIXED,37.37036978808,126.72474421663,11.9786,22.3000,0.0047,0.0067,-0.0013,-0.928872282,-0.553697903,17.517066797,0.2114,0.1694,0.2805,0.0344,0.0343,0.0312,0.0907,0.0906,5.0009,0f000005,0*82370f01\n\t", "INSPVAXA,USB3,0,48.0,FINESTEERING,2107,282544.300,02000000,471d,15824;INS_ALIGNMENT_COMPLETE,INS_RTKFIXED,37.37036978718,126.72474422252,11.9791,22.3000,0.0050,0.0075,-0.0009,-0.927752537,-0.554071617,17.520424988,0.2100,0.1688,0.2784,0.0344,0.0343,0.0312,0.0907,0.0906,5.0016,0f000005,0*49ddb25e\n\t", "INSPVAXA,USB3,0,53.5,FINESTEERING,2107,282545.300,02000000,471d,15824;INS_ALIGNMENT_COMPLETE,INS_RTKFIXED,37.37036978780,126.72474423597,11.9800,22.3000,0.0057,0.0083,-0.0009,-0.928955270,-0.556659183,17.532369164,0.2088,0.1684,0.2765,0.0344,0.0343,0.0312,0.0907,0.0906,5.0023,0f000005,0*6d6cecb2\n\t", "INSPVAXA,USB3,0,53.5,FINESTEERING,2107,282545.800,02000000,471d,15824;INS_ALIGNMENT_COMPLETE,INS_RTKFIXED,37.37036979074,126.72474423499,11.9811,22.3000,0.0059,0.0071,-0.0001,-0.929937499,-0.555084001,17.534967514,0.2088,0.1684,0.2765,0.0344,0.0343,0.0312,0.0907,0.0906,5.0023,0f000005,0*3f4b51d6\n\t", "INSPVAXA,USB3,0,52.0,FINESTEERING,2107,282546.300,02000000,471d,15824;INS_ALIGNMENT_COMPLETE,INS_RTKFIXED,37.37036979075,126.72474423167,11.9818,22.3000,0.0060,0.0065,0.0000,-0.930882375,-0.556370443,17.539693499,0.2078,0.1680,0.2748,0.0344,0.0343,0.0312,0.0907,0.0906,5.0033,0f000005,0*966ea92a\n\t", "INSPVAXA,USB3,0,52.0,FINESTEERING,2107,282546.800,02000000,471d,15824;INS_ALIGNMENT_COMPLETE,INS_RTKFIXED,37.37036979117,126.72474423599,11.9822,22.3000,0.0059,0.0073,0.0004,-0.930733937,-0.558015059,17.542914656,0.2078,0.1680,0.2748,0.0344,0.0343,0.0312,0.0907,0.0906,5.0033,0f000005,0*c41d3119\n\t", "INSPVAXA,USB3,0,48.0,FINESTEERING,2107,282547.300,02000000,471d,15824;INS_ALIGNMENT_COMPLETE,INS_RTKFIXED,37.37036978952,126.72474423883,11.9826,22.3000,0.0057,0.0074,0.0003,-0.934085906,-0.556515155,17.545794834,0.2070,0.1677,0.2732,0.0344,0.0343,0.0312,0.0907,0.0906,5.0042,0f000005,0*0a93c56e\n
